vi "Create MQTT Server.vi"(5 "Server in":refnum<class "Server.lvclass">) -> (3 "MQTT Server":refnum<class "Server.lvclass">)   [LabVIEW 2013, in "MQTT Server.lvlib"]
uses:
  Server/MQTT Server.lvlib
  Server/Server class/Server.lvclass
panel:
  out "error out":errorcluster
  in  "error in (no error)":errorcluster
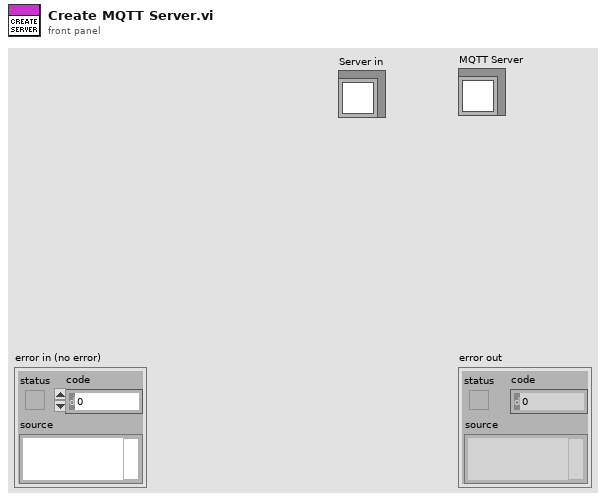
[diagram p1: front panel]
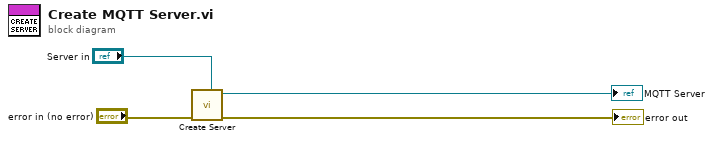
[diagram p0: block diagram]
diagram:
  n1 = call "Create Server.vi"("Server in"="Server in", "error in (no error)"="error in (no error)") -> ("error out"=→"error out":errorcluster, "Server"=→"MQTT Server":refnum<class "Server.lvclass">)  [unwired: 8 in]
